vi "FFTCalc_SubVI.vi"(8 "error in (no error)":errorcluster, 11 "Waveform":waveform(dbl)) -> (0 "error out":errorcluster, 3 "Power Spectrum / PSD":cluster{"f0":dbl, "df":dbl, "magnitude":dbl[]})   [LabVIEW 2019]
doc: "This SubVI calculates the FFT of the waveform.\n\nIN: Waveform; Error in;\nOUT: Power Spectrum; Error out;"
uses:
  <vilib>/measure/NI_MAPro.lvlib
  <vilib>/measure/maspectr.llb/FFT Power Spectrum and PSD for 1 Chan.vi
  <vilib>/Analysis/4window.llb/windowTd.ctl
  <vilib>/Analysis/NI_AALPro.lvlib
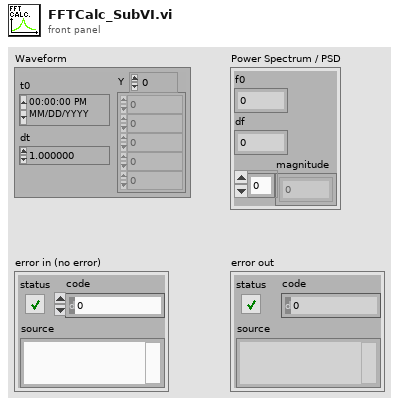
[diagram p1: front panel]
types:
  T1 = typedef "NI_AALPro.lvlib/windowTd.ctl" = u32
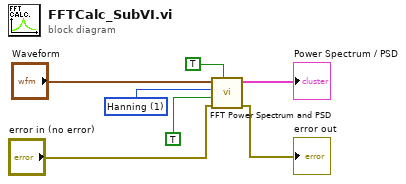
[diagram p0: block diagram]
diagram:
  w3 = T1 1 items=["Rectangle"=0, "Hanning"=1, "Hamming"=2, "Blackman-Harris"=3, "Exact Blackman"=4, "Blackman"=5, "Flat Top"=6, "4 Term B-Harris "=7, "7 Term B-Harris"=8, "Low Sidelobe"=9, "Blackman Nuttall"=11, "Triangle"=30, "Bartlett-Hanning"=31, "Bohman"=32, "Parzen"=33, "Welch"=34, "Kaiser"=60, "Dolph-Chebyshev"=61, "Gaussian"=62] ("window")
  n1 = call-poly <vilib>:"FFT Power Spectrum and PSD.vi"("restart averaging (F)"=TRUE, "error in (no error)"="error in (no error)", "dB On (F)"=TRUE, "window"=w3, "time signal"="Waveform") -> ("error out"=→"error out":errorcluster, "Power Spectrum / PSD"=→"Power Spectrum / PSD":cluster{"f0":dbl, "df":dbl, "magnitude":dbl[]})  [unwired: 3 in, 2 out]
